vi "Test Sleep FTE.vi"() -> ()   [LabVIEW 2021]
uses:
  System Time/LabVIEW Time to TAI Time.vi
  SubVIs/Add Error.vi
  Errors/Append Error Location.vi
  Time_CIF_U.lvlib
panel:
  out "Sleep Errors":i64[](array[numeric])
  out "status":string
  out "pass":bool
  out "error out":errorcluster
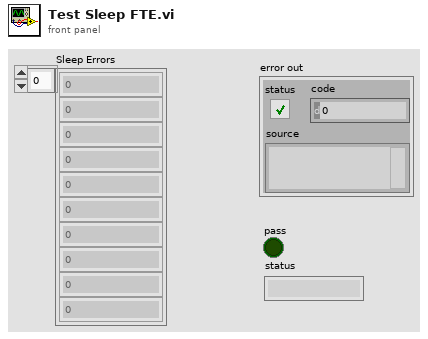
[diagram p1: front panel]
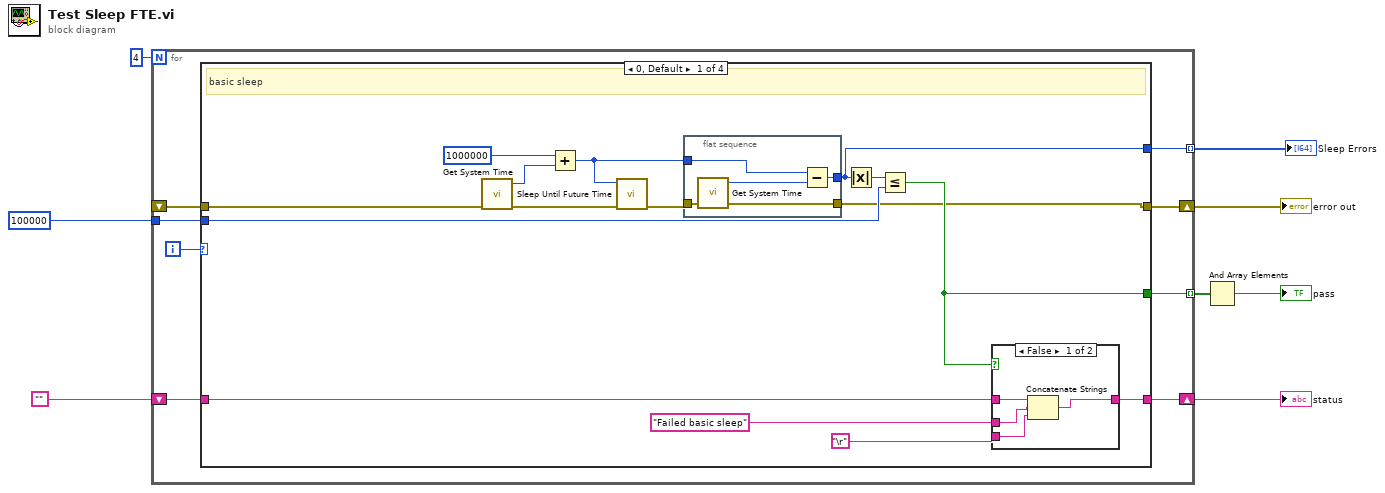
[diagram p0: block diagram]
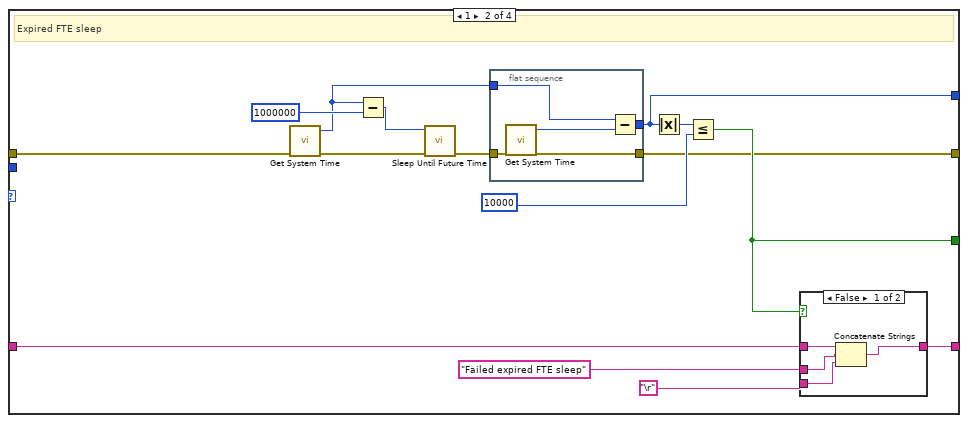
[diagram p3: hidden frame]
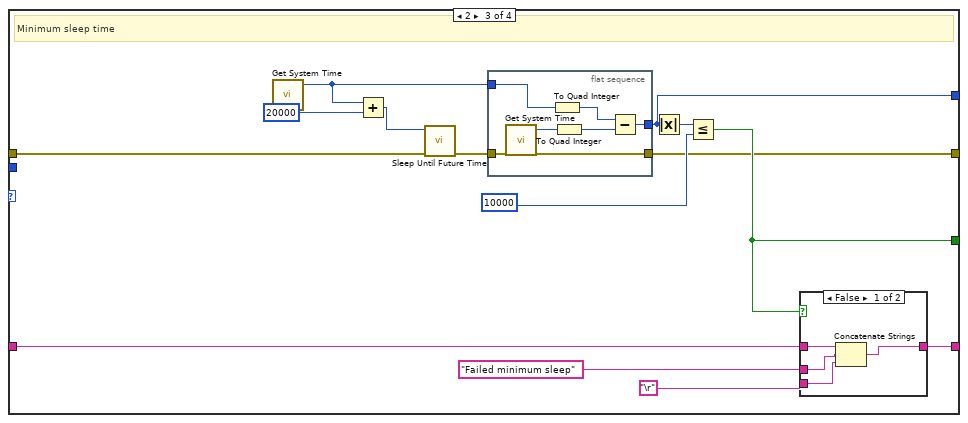
[diagram p5: hidden frame]
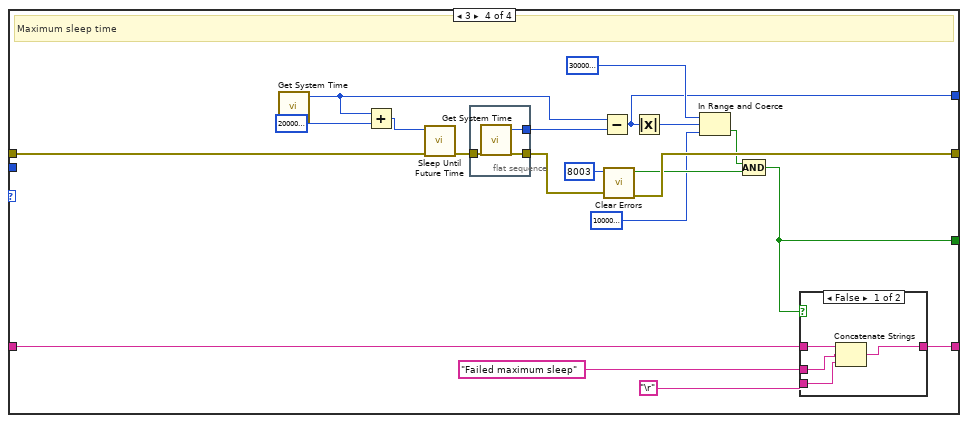
[diagram p7: hidden frame]
diagram:
  n1 = for {
    N: 4 -> [_]
    tunnel: [w16] -> w2 mode=indexing
    shift-right: [w13] -> w6
    shift-left: "" -> [w14]
    tunnel: i64 100000 ("y") -> [w12]
    shift-right: [w11] -> w4
    shift-left: _ -> [w10]
    tunnel: [w9] -> w3 mode=indexing
    i -> [w15]
    n2 = case shown="0, Default" w15 {
      tunnel: [w23 w48 w71 w99] -> w16
      tunnel: w14 -> [w30 w53 w76 w107]
      tunnel: [w29 w52 w75 w106] -> w13
      tunnel: w12 -> [w24 _ _ _]
      tunnel: [w20 w44 w66 w101] -> w11
      tunnel: w10 -> [w22 w43 w68 w95]
      tunnel: [w18 w41 w64 w89] -> w9
      frame 0, Default {
        # "basic sleep"
        n3 = call "Get System Time.vi"() -> ("Time (ns)"=w26:i64)  [unwired: 5 in]
        n4 = Add(x=i64 1000000, y=w26) -> (x+y=w19:i64)
        n5 = call "Sleep Until Future Time.vi"("error in (no error)"=w22, "Wake Time (ns)"=w19) -> ("error out"=w21:errorcluster)  [unwired: 8 in, 1 out]
        n6 = flat-sequence {
          tunnel: [w34] -> w18
          tunnel: w19 -> [w32]
          tunnel: w21 -> [w31]
          tunnel: [w31] -> w20
          frame #0 {
            n7 = call "Get System Time.vi"() -> ("Time (ns)"=w33:i64)  [unwired: 5 in]
            n8 = Subtract(x=w32, y=w33) -> (x-y=w34:i64)
          }
        }
        n9 = Absolute Value(x=w18) -> (abs(x)=w17:i64)
        n10 = Less Or Equal?(x=w17, y=w24) -> (x <= y?=w23:bool)
        n11 = case shown="False" w23 {
          tunnel: w30 -> [w38 w39]
          tunnel: [w35 w39] -> w29
          tunnel: "Failed basic sleep" -> [w37 _]
          tunnel: "\r" -> [w36 _]
          frame False {
            n12 = Concatenate Strings(w38, w37, w36) -> (w35:string)
          }
          frame True {
          }
        }
      }
      frame 1 {
        # "Expired FTE sleep"
        n13 = call "Get System Time.vi"() -> ("Time (ns)"=w47:i64)  [unwired: 5 in]
        n14 = Subtract(x=w47, y=i64 1000000 ("x")) -> (x-y=w42:i64)
        n15 = call "Sleep Until Future Time.vi"("error in (no error)"=w43, "Wake Time (ns)"=w42) -> ("error out"=w45:errorcluster)  [unwired: 8 in, 1 out]
        n16 = flat-sequence {
          tunnel: [w57] -> w41
          tunnel: w47 -> [w55]
          tunnel: w45 -> [w54]
          tunnel: [w54] -> w44
          frame #0 {
            n17 = call "Get System Time.vi"() -> ("Time (ns)"=w56:i64)  [unwired: 5 in]
            n18 = Subtract(x=w55, y=w56) -> (x-y=w57:i64)
          }
        }
        n19 = Absolute Value(x=w41) -> (abs(x)=w40:i64)
        n20 = Less Or Equal?(x=w40, y=i64 10000) -> (x <= y?=w48:bool)
        n21 = case shown="False" w48 {
          tunnel: w53 -> [w61 w62]
          tunnel: [w58 w62] -> w52
          tunnel: "Failed expired FTE sleep" -> [w60 _]
          tunnel: "\r" -> [w59 _]
          frame False {
            n22 = Concatenate Strings(w61, w60, w59) -> (w58:string)
          }
          frame True {
          }
        }
      }
      frame 2 {
        # "Minimum sleep time"
        n23 = call "Get System Time.vi"() -> ("Time (ns)"=w70:i64)  [unwired: 5 in]
        n24 = Add(x=w70, y=i64 20000 ("x")) -> (x+y=w65:i64)
        n25 = call "Sleep Until Future Time.vi"("error in (no error)"=w68, "Wake Time (ns)"=w65) -> ("error out"=w67:errorcluster)  [unwired: 8 in, 1 out]
        n26 = flat-sequence {
          tunnel: [w79] -> w64
          tunnel: w70 -> [w78]
          tunnel: w67 -> [w77]
          tunnel: [w77] -> w66
          frame #0 {
            n27 = call "Get System Time.vi"() -> ("Time (ns)"=w82:i64)  [unwired: 5 in]
            n28 = To Quad Integer(1:w78) -> (0:w81:i64)
            n29 = To Quad Integer(1:w82) -> (0:w80:i64)
            n30 = Subtract(x=w81, y=w80) -> (x-y=w79:i64)
          }
        }
        n31 = Absolute Value(x=w64) -> (abs(x)=w63:i64)
        n32 = Less Or Equal?(x=w63, y=i64 10000) -> (x <= y?=w71:bool)
        n33 = case shown="False" w71 {
          tunnel: w76 -> [w86 w87]
          tunnel: [w83 w87] -> w75
          tunnel: "Failed minimum sleep" -> [w85 _]
          tunnel: "\r" -> [w84 _]
          frame False {
            n34 = Concatenate Strings(w86, w85, w84) -> (w83:string)
          }
          frame True {
          }
        }
      }
      frame 3 {
        # "Maximum sleep time"
        n35 = call "Get System Time.vi"() -> ("Time (ns)"=w91:i64)  [unwired: 5 in]
        n36 = Add(x=w91, y=i64 2000000000 ("x")) -> (x+y=w90:i64)
        n37 = call "Sleep Until Future Time.vi"("error in (no error)"=w95, "Wake Time (ns)"=w90) -> ("error out"=w94:errorcluster)  [unwired: 8 in, 1 out]
        n38 = flat-sequence {
          tunnel: [w109] -> w92
          tunnel: w94 -> [w108]
          tunnel: [w108] -> w93
          frame #0 {
            n39 = call "Get System Time.vi"() -> ("Time (ns)"=w109:i64)  [unwired: 5 in]
          }
        }
        n40 = Subtract(x=w91, y=w92) -> (x-y=w89:i64)
        n41 = call <vilib>:"Clear Errors.vi"("error in (no error)"=w93, "specific error code to clear (0: all)"=8003) -> ("error out"=w101:errorcluster, "specific error cleared?"=w100:bool)  [unwired: 4 in]
        n42 = Absolute Value(x=w89) -> (abs(x)=w88:i64)
        n43 = In Range and Coerce(upper limit=i64 300000000 ("y"), x=w88, lower limit=i64 100000000 ("y")) -> (In Range?=w98:bool)  [unwired: 1 out]
        n44 = Compound Arithmetic op=AND(w98, w100) -> (w99:bool)
        n45 = case shown="False" w99 {
          tunnel: w107 -> [w113 w114]
          tunnel: [w110 w114] -> w106
          tunnel: "Failed maximum sleep" -> [w112 _]
          tunnel: "\r" -> [w111 _]
          frame False {
            n46 = Concatenate Strings(w113, w112, w111) -> (w110:string)
          }
          frame True {
          }
        }
      }
    }
  }
  "error out" <- w4
  "status" <- w6
  "Sleep Errors" <- w3
  n47 = And Array Elements(Boolean array=w2) -> (logical AND=→"pass":bool)
